vi "Red Rack Enclosure test.vi"() -> (0 "Red Rack Enclosure OK":bool)   [LabVIEW 2015]
uses:
  <vilib>/DAQmx/read.llb/DAQmx Read (Digital Bool 1Line 1Point).vi
  <vilib>/DAQmx/miscellaneous.llb/DAQmx Fill In Error Info.vi
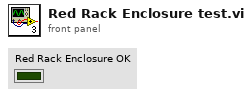
[diagram p1: front panel]
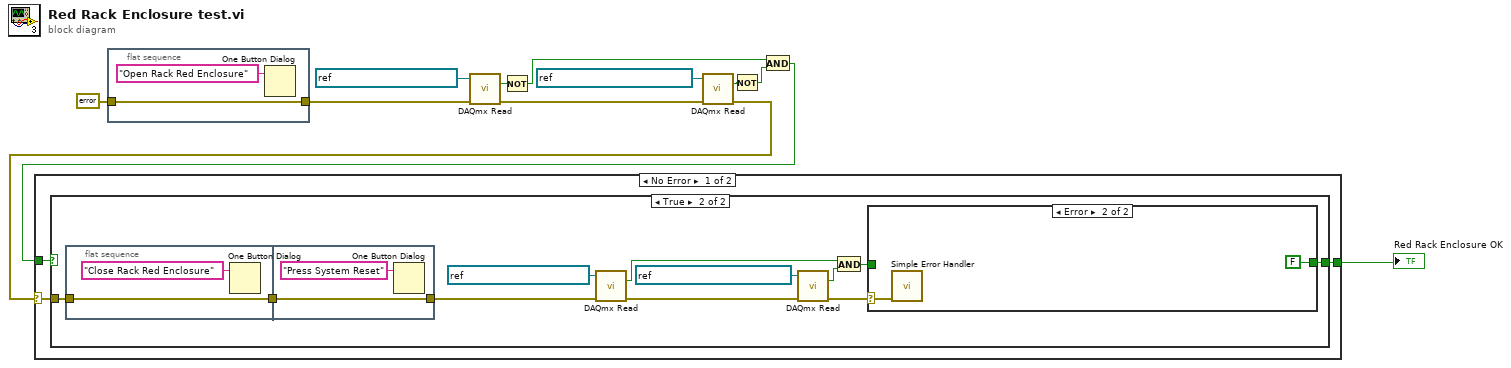
[diagram p0: block diagram]
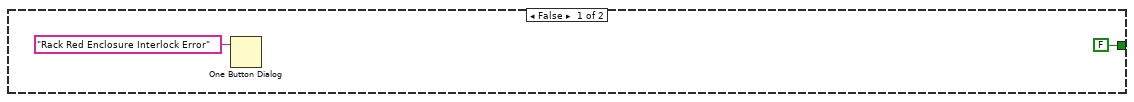
[diagram p2: hidden frame]
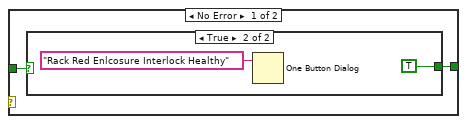
[diagram p3: hidden frame]
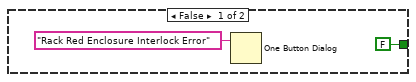
[diagram p4: hidden frame]
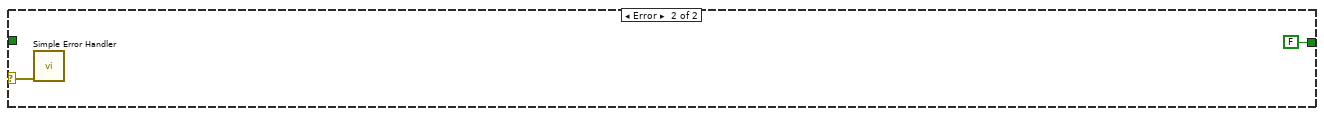
[diagram p5: hidden frame]
diagram:
  n1 = flat-sequence {
    tunnel: errorcluster {"status"=FALSE, "code"=0, "source"=""} ("error constant") -> [w13]
    tunnel: [w13] -> w4
    frame #0 {
      n2 = One Button Dialog(message="Open Rack Red Enclosure") -> ()  [unwired: 1 in, 1 out]
    }
  }
  n3 = call-poly <vilib>:"DAQmx Read.vi"("task/channels in"=refnum<k21> "DI1 Safety System trip" ("DAQmx Global Channel"), "error in"=w4) -> ("data"=w5:bool, "error out"=w8:errorcluster)  [unwired: 11 in, 1 out]
  n4 = Not(x=w5) -> (.not. x?=w10:bool)
  n5 = call-poly <vilib>:"DAQmx Read.vi"("task/channels in"=refnum<k21> "DI5 Dump Switch mimic" ("DAQmx Global Channel"), "error in"=w8) -> ("data"=w6:bool, "error out"=w11:errorcluster)  [unwired: 11 in, 1 out]
  n6 = Not(x=w6) -> (.not. x?=w9:bool)
  n7 = And(x=w10, y=w9) -> (x .and. y?=w12:bool)
  n8 = case shown="No Error" w11 {
    selector: w11 -> [w16 w44]
    tunnel: w12 -> [w17 _]
    tunnel: [w15 FALSE] -> w1
    frame No Error {
      n9 = case shown="True" w17 {
        tunnel: w16 -> [_ w29]
        tunnel: [FALSE w20] -> w15
        frame False {
          n10 = One Button Dialog(message="Rack Red Enclosure Interlock Error") -> ()  [unwired: 1 in, 1 out]
        }
        frame True {
          n11 = flat-sequence {
            tunnel: w29 -> [w39]
            tunnel: [w39] -> w30
            tunnel: [w42] -> w21
            tunnel: w30 -> [w42]
            frame #0 {
              n12 = One Button Dialog(message="Close Rack Red Enclosure") -> ()  [unwired: 1 in, 1 out]
            }
            frame #1 {
              n13 = One Button Dialog(message="Press System Reset") -> ()  [unwired: 1 in, 1 out]
            }
          }
          n14 = call-poly <vilib>:"DAQmx Read.vi"("task/channels in"=refnum<k21> "DI1 Safety System trip" ("DAQmx Global Channel"), "error in"=w21) -> ("data"=w25:bool, "error out"=w28:errorcluster)  [unwired: 11 in, 1 out]
          n15 = call-poly <vilib>:"DAQmx Read.vi"("task/channels in"=refnum<k21> "DI5 Dump Switch mimic" ("DAQmx Global Channel"), "error in"=w28) -> ("data"=w24:bool, "error out"=w22:errorcluster)  [unwired: 11 in, 1 out]
          n16 = And(x=w25, y=w24) -> (x .and. y?=w23:bool)
          n17 = case shown="Error" w22 {
            selector: w22 -> [_ w37]
            tunnel: w23 -> [w32 _]
            tunnel: [w31 FALSE] -> w20
            frame No Error {
              n18 = case shown="True" w32 {
                tunnel: [FALSE TRUE] -> w31
                frame False {
                  n19 = One Button Dialog(message="Rack Red Enclosure Interlock Error") -> ()  [unwired: 1 in, 1 out]
                }
                frame True {
                  n20 = One Button Dialog(message="Rack Red Enlcosure Interlock Healthy") -> ()  [unwired: 1 in, 1 out]
                }
              }
            }
            frame Error {
              n21 = call <vilib>:"Simple Error Handler.vi"("error in (no error)"=w37) -> ()  [unwired: 4 in, 5 out]
            }
          }
        }
      }
    }
    frame Error {
      n22 = call <vilib>:"Simple Error Handler.vi"("error in (no error)"=w44) -> ()  [unwired: 4 in, 5 out]
    }
  }
  "Red Rack Enclosure OK" <- w1
